vi "Get Modifier from Key Event.vi"(0 "Modifiers":T1) -> (1 "Modifiers":T2[](array[typedef]), 2 "Modifiers Concatenated":string)   [LabVIEW 2021, in "Seq Edit Quick Drop.lvlib"]
uses:
  Seq Edit Quick Drop.lvlib
  Modifiers.ctl
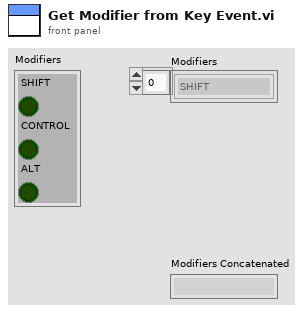
[diagram p1: front panel]
types:
  T1 = cluster{"SHIFT":bool, "CONTROL":bool, "ALT":bool}
  T2 = typedef "Seq Edit Quick Drop.lvlib/Modifiers.ctl" = enum16{"SHIFT", "CTRL", "ALT"}
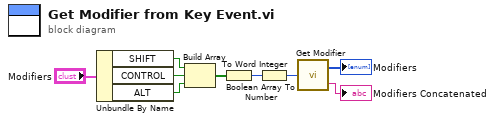
[diagram p0: block diagram]
diagram:
  n1 = Unbundle By Name("Modifiers") -> ("SHIFT"=w9:bool, "CONTROL"=w8:bool, "ALT"=w7:bool)
  n2 = Build Array(w9, w8, w7) -> (w6:bool[])
  n3 = Boolean Array To Number(Boolean array=w6) -> (number=w5:u32)
  n4 = To Word Integer(number=w5) -> (16bit integer=w4:i16)
  n5 = call "Get Modifier.vi"("Modifier Code"=w4) -> ("Modifiers"=→"Modifiers":T2[], "Modifiers Concatenated"=→"Modifiers Concatenated":string)
